vi "test4.vi"() -> ()   [LabVIEW 2013]
panel:
  out "read message":string
  out "handle":i32
  in  "file path":string="\\\\.\\Pipe\\MyNamedPipe"
  out "error out":errorcluster
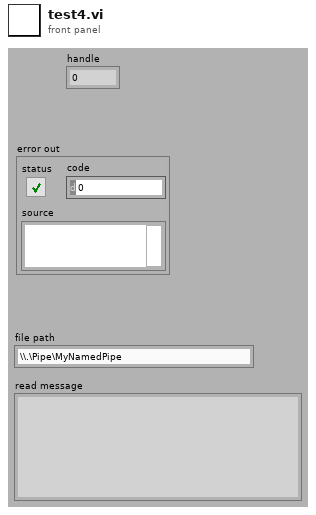
[diagram p1: front panel]
types:
  T1 = enum16{"CREATE_NEW", "CREATE_ALWAYS", "OPEN_EXISTING", "OPEN_ALWAYS", "TRUNCATE_EXISTING"}
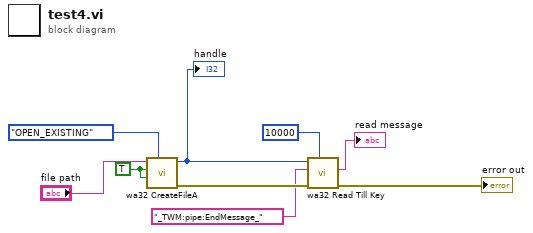
[diagram p0: block diagram]
diagram:
  w5 = TRUE ("read")
  n1 = call "wa32 CreateFileA.vi"("creation dispozition"=T1."OPEN_EXISTING", "write"=w5, "read"=w5, "file path"="file path") -> ("error out"=w9:errorcluster, "handle"=w8:i32)  [unwired: 6 in]
  "handle" <- w8
  n2 = call "wa32 Read Till Key.vi"("timeout [ms] (1000)"=10000, "error in"=w9, "key string"="_TWM:pipe:EndMessage_", "handle"=w8) -> ("error out"=→"error out":errorcluster, "read message"=→"read message":string)  [unwired: 5 in, 1 out]
